vi "Read Test Sequence.vi"(8 "error in (no error)":errorcluster, 11 "NI DAQmx in":refnum<class "NI DAQmx.lvclass">) -> (0 "error out":errorcluster, 2 "Test Sequence":T1, 3 "NI DAQmx out":refnum<class "NI DAQmx.lvclass">)   [LabVIEW 2020, in "NI DAQmx.lvclass"]
uses:
  NI DAQmx.lvclass
  NI DAQmx.lvclass/NI DAQmx.ctl
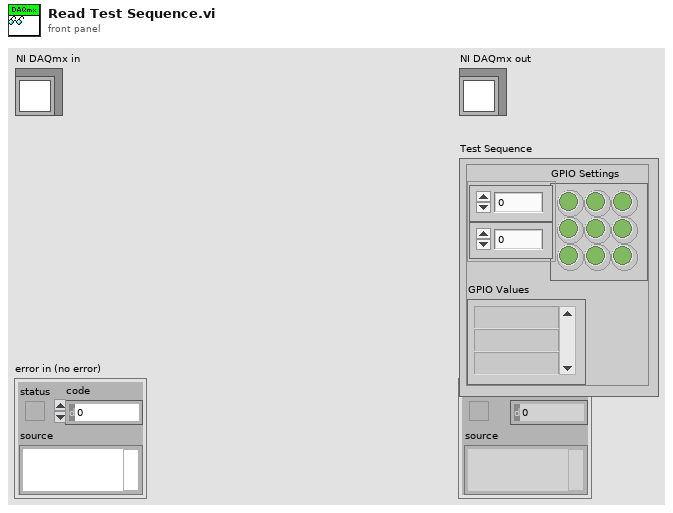
[diagram p1: front panel]
types:
  T1 = cluster{"GPIO Settings":bool[][], "GPIO Values":string[]}
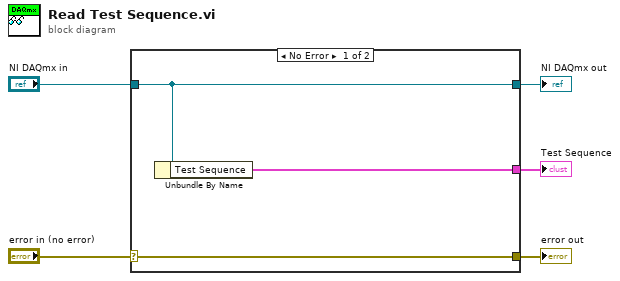
[diagram p0: block diagram]
diagram:
  n1 = case shown="No Error" "error in (no error)" {
    selector: "error in (no error)" -> [w8 w9]
    tunnel: [w8 w9] -> w4
    tunnel: [w7 w10] -> w2
    tunnel: "NI DAQmx in" -> [w7 w10]
    tunnel: [w6 _] -> w1
    frame No Error {
      n2 = Unbundle By Name(w7) -> ("Test Sequence"=w6:T1)
    }
    frame Error {
    }
  }
  "error out" <- w4
  "NI DAQmx out" <- w2
  "Test Sequence" <- w1
